vi "Set PN.vi"(8 "error in (no error)":errorcluster caption="entrée d'erreur (pas d'erreur)", 10 "PN":string, 11 "Firebase Recovery_SN en entrée":refnum<class "Firebase Recovery_SN.lvclass">) -> (0 "error out":errorcluster caption="sortie d'erreur", 3 "Firebase Recovery_SN en sortie":refnum<class "Firebase Recovery_SN.lvclass">)   [LabVIEW 2020, in "Library Instrument & Equipement.lvlib" / "Library FireBase.lvlib" / "Firebase Recovery_SN.lvclass"]
uses:
  Firebase Recovery_SN.lvclass
  Firebase Recovery_SN.lvclass/Firebase Recovery_SN.ctl
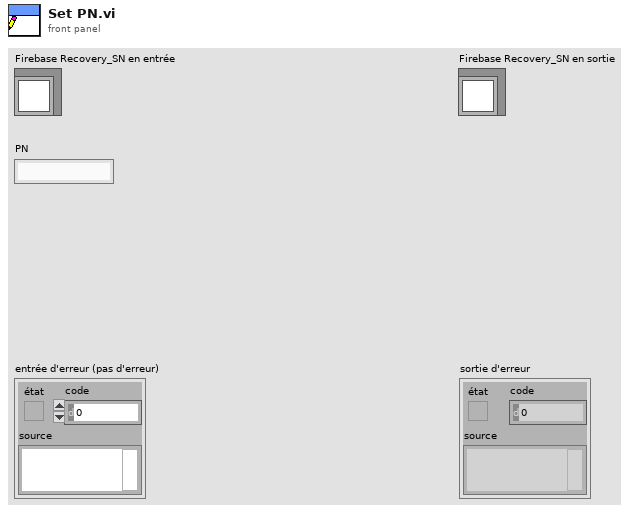
[diagram p1: front panel]
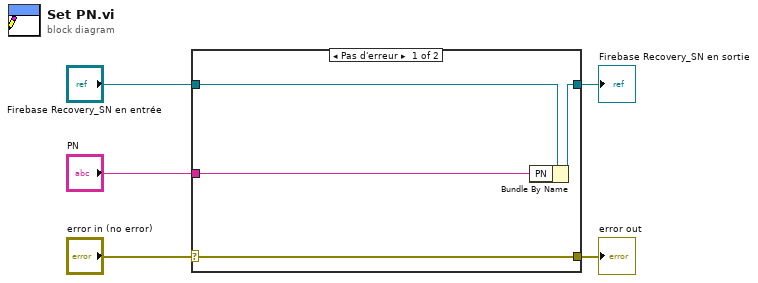
[diagram p0: block diagram]
diagram:
  n1 = case shown="Pas d'erreur" "error in (no error)" {
    selector: "error in (no error)" -> [w9 w10]
    tunnel: [w9 w10] -> w4
    tunnel: [w7 w11] -> w2
    tunnel: "Firebase Recovery_SN en entrée" -> [w8 w11]
    tunnel: "PN" -> [w6 _]
    frame No Error {
      n2 = Bundle By Name(cluster=w8, "PN"=w6) -> (w7:refnum<class "Firebase Recovery_SN.lvclass">)
    }
    frame Error {
    }
  }
  "error out" <- w4
  "Firebase Recovery_SN en sortie" <- w2
